vi "update.vi"(8 "error in (no error)":errorcluster, 10 "model":refnum<class "Model.lvclass">, 11 "EndingCycleState in":refnum<class "EndingCycleState.lvclass">) -> (0 "error out":errorcluster, 2 "model 2":refnum<class "Model.lvclass">, 3 "EndingCycleState out":refnum<class "EndingCycleState.lvclass">)   [LabVIEW 2013, in "EndingCycleState.lvclass"]
uses:
  EndingCycleState.lvclass
  Model/Model/Model.lvclass
  AutomatedMotionState/AutomatedMotionState.lvclass
  Typedefs/StateSelector.ctl
  Typedefs/M2AADTTypedefs.lvlib
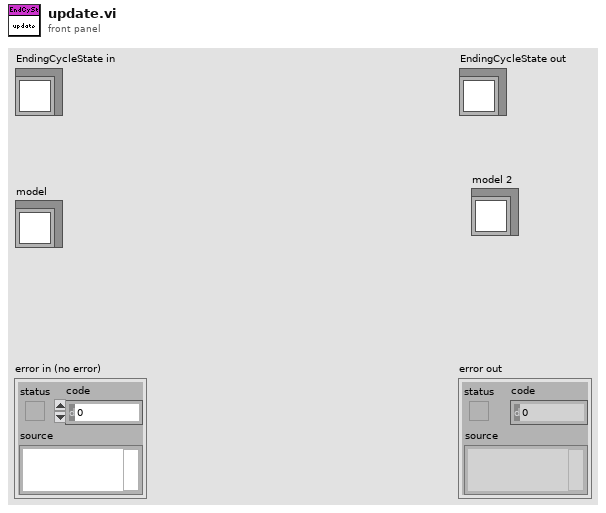
[diagram p1: front panel]
types:
  T1 = typedef "M2AADTTypedefs.lvlib/StateSelector.ctl" = enum16{"EndingCycleState", "FaultState", "InteractiveMotionState", "MovingToNewForceState", "OffState", "PausingState", "StandbyState", "StoppedState"}
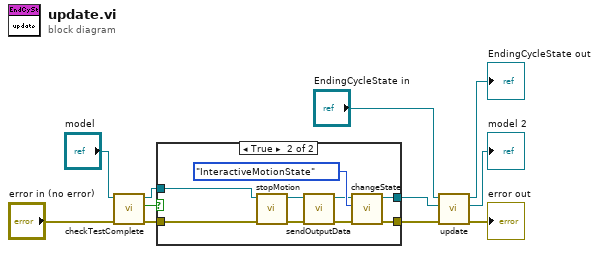
[diagram p0: block diagram]
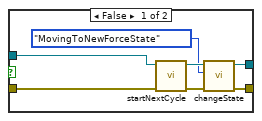
[diagram p2: hidden frame]
diagram:
  n1 = call "checkTestComplete.vi"("error in (no error)"="error in (no error)", "Model in"="model") -> ("error out"=w4:errorcluster, "testCompleteIsTrue"=w1:bool, "Model out"=w6:refnum<class "Model.lvclass">)  [unwired: 7 in]
  n2 = case shown="True" w1 {
    tunnel: w6 -> [w18 w27]
    tunnel: w4 -> [w15 w25]
    tunnel: [w13 w24] -> w3
    tunnel: [w16 w23] -> w2
    frame False {
      n3 = call "startNextCycle.vi"("error in (no error)"=w15, "Model in"=w18) -> ("error out"=w14:errorcluster, "Model out"=w17:refnum<class "Model.lvclass">)  [unwired: 8 in]
      n4 = call "changeState.vi"("error in (no error)"=w14, "State:"=StateSelector."MovingToNewForceState", "Model in"=w17) -> ("error out"=w13:errorcluster, "Model out"=w16:refnum<class "Model.lvclass">)  [unwired: 7 in]
    }
    frame True {
      n5 = call "stopMotion.vi"("error in (no error)"=w25, "Model in"=w27) -> ("error out"=w21:errorcluster, "Model out"=w22:refnum<class "Model.lvclass">)  [unwired: 8 in]
      n6 = call "sendOutputData.vi"("error in (no error)"=w21, "Model in"=w22) -> ("error out"=w20:errorcluster, "Model out"=w19:refnum<class "Model.lvclass">)  [unwired: 8 in]
      n7 = call "changeState.vi"("error in (no error)"=w20, "State:"=StateSelector."InteractiveMotionState", "Model in"=w19) -> ("error out"=w24:errorcluster, "Model out"=w23:refnum<class "Model.lvclass">)  [unwired: 7 in]
    }
  }
  n8 = call-parent "update.vi"("error in (no error)"=w3, "model"=w2, "ControlledMotionState in"="EndingCycleState in") -> ("error out"=→"error out":errorcluster, "model 2"=→"model 2":refnum<class "Model.lvclass">, "ControlledMotionState out"=→"EndingCycleState out":refnum<class "EndingCycleState.lvclass">)  [unwired: 6 in]
